vi "全局 CODMn.vi"() -> ()   [LabVIEW 2016]
panel:
  in  "CODMn":string[][](array[string])
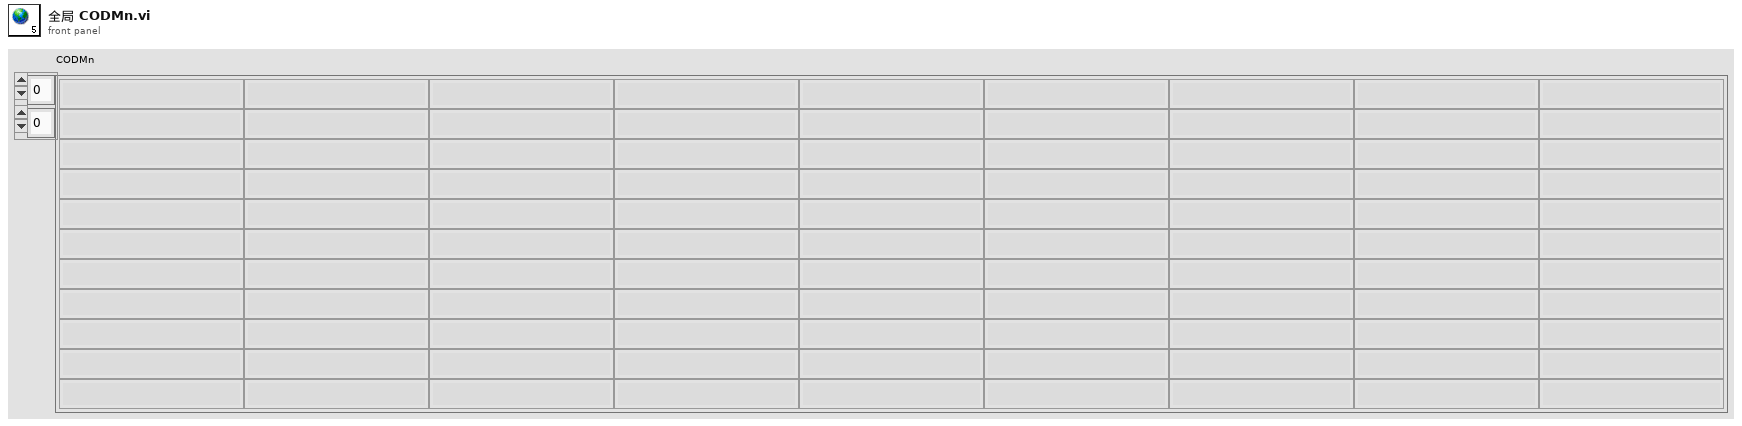
[diagram p1: front panel]
diagram:
